vi "Get Font.vi"(0 "Font":refnum<class "Font Class.lvclass">, 7 "Font IN":T1={"Name"="STFANGSO", "Size"=12.0, "Color"=0, "Style"={"Bold"=FALSE, "Italic"=FALSE, "Underline"=FALSE, "Strikeout"=FALSE}, "Type"={"Type&direction"=enum."Select", "Embedded"=FALSE, "Encoding"=""}}, 11 "error in (no error)":errorcluster) -> (4 "Font duplicate":refnum<class "Font Class.lvclass">, 6 "Font":refnum<k24>, 8 "Font OUT":T1={"Name"="STFANGSO", "Size"=12.0, "Color"=0, "Style"={"Bold"=FALSE, "Italic"=FALSE, "Underline"=FALSE, "Strikeout"=FALSE}, "Type"={"Type&direction"=enum."Select", "Embedded"=FALSE, "Encoding"=""}}, 10 "Font Size":T2=12.0, 15 "error out":errorcluster)   [LabVIEW 2020, in "Exaprom PDF.lvlib" / "Font Class.lvclass"]
doc: "Version 1.0\nDeveloped by Jean-Marc Simard\nCopyright © 2012, Exaprom Inc.\nAll rights reserved.\nLicense: BSD\n\nWith iTextSharp 4.1.6 (http://itextsharp.sourceforge.net)\nunder Mozilla Public License Version 1.1\n(http://www.mozilla.org/MPL/MPL-1.1.html)"
uses:
  <userlib>/labview-PDF-writer-master/LV Class/Fonts Class/Font Class.lvclass
  <userlib>/labview-PDF-writer-master/Controls/Font Controls/Font complete cluster.ctl
  <userlib>/labview-PDF-writer-master/Controls/Font Controls/Font size.ctl
  <userlib>/labview-PDF-writer-master/Controls/Font Controls/Font color.ctl
  <userlib>/labview-PDF-writer-master/Controls/Font Controls/Type and encoding.ctl
  <userlib>/labview-PDF-writer-master/Controls/Text Controls/Unicode/Type and run direction.ctl
  C:/Program Files (x86)/National Instruments/LabVIEW 2020/user.lib/labview-PDF-writer-master/DLL/itextsharp.dll
  DLL/itextsharp.dll
  <userlib>/labview-PDF-writer-master/LV Class/Fonts Class/Font Class.lvclass/Font Class.ctl
  <userlib>/labview-PDF-writer-master/Exaprom PDF.lvlib
panel:
  out "NOT_EMBEDDED":bool
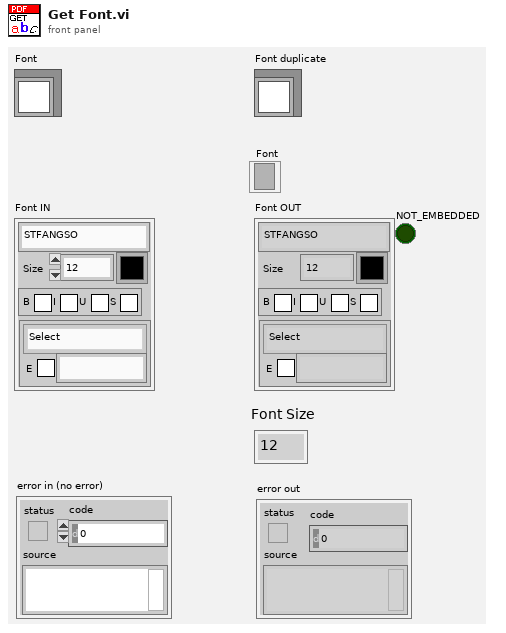
[diagram p1: front panel]
types:
  T1 = typedef "Exaprom PDF.lvlib/Font complete cluster.ctl" = cluster{"Name":string, "Size":T2, "Color":T3, "Style":cluster{"Bold":bool, "Italic":bool, "Underline":bool, "Strikeout":bool}, "Type":T4}
  T2 = typedef "Exaprom PDF.lvlib/Font size.ctl" = sgl
  T3 = typedef "Exaprom PDF.lvlib/Font color.ctl" = u32
  T4 = typedef "Exaprom PDF.lvlib/Type and encoding.ctl" = cluster{"Type&direction":T5, "Embedded":bool, "Encoding":string}
  T5 = typedef "Exaprom PDF.lvlib/Type and run direction.ctl" = enum16{"Select", "ASCII", "UTF-16", "UTF-16 (default)", "UTF-16 (LTR)", "UTF-16 (RTL)"}
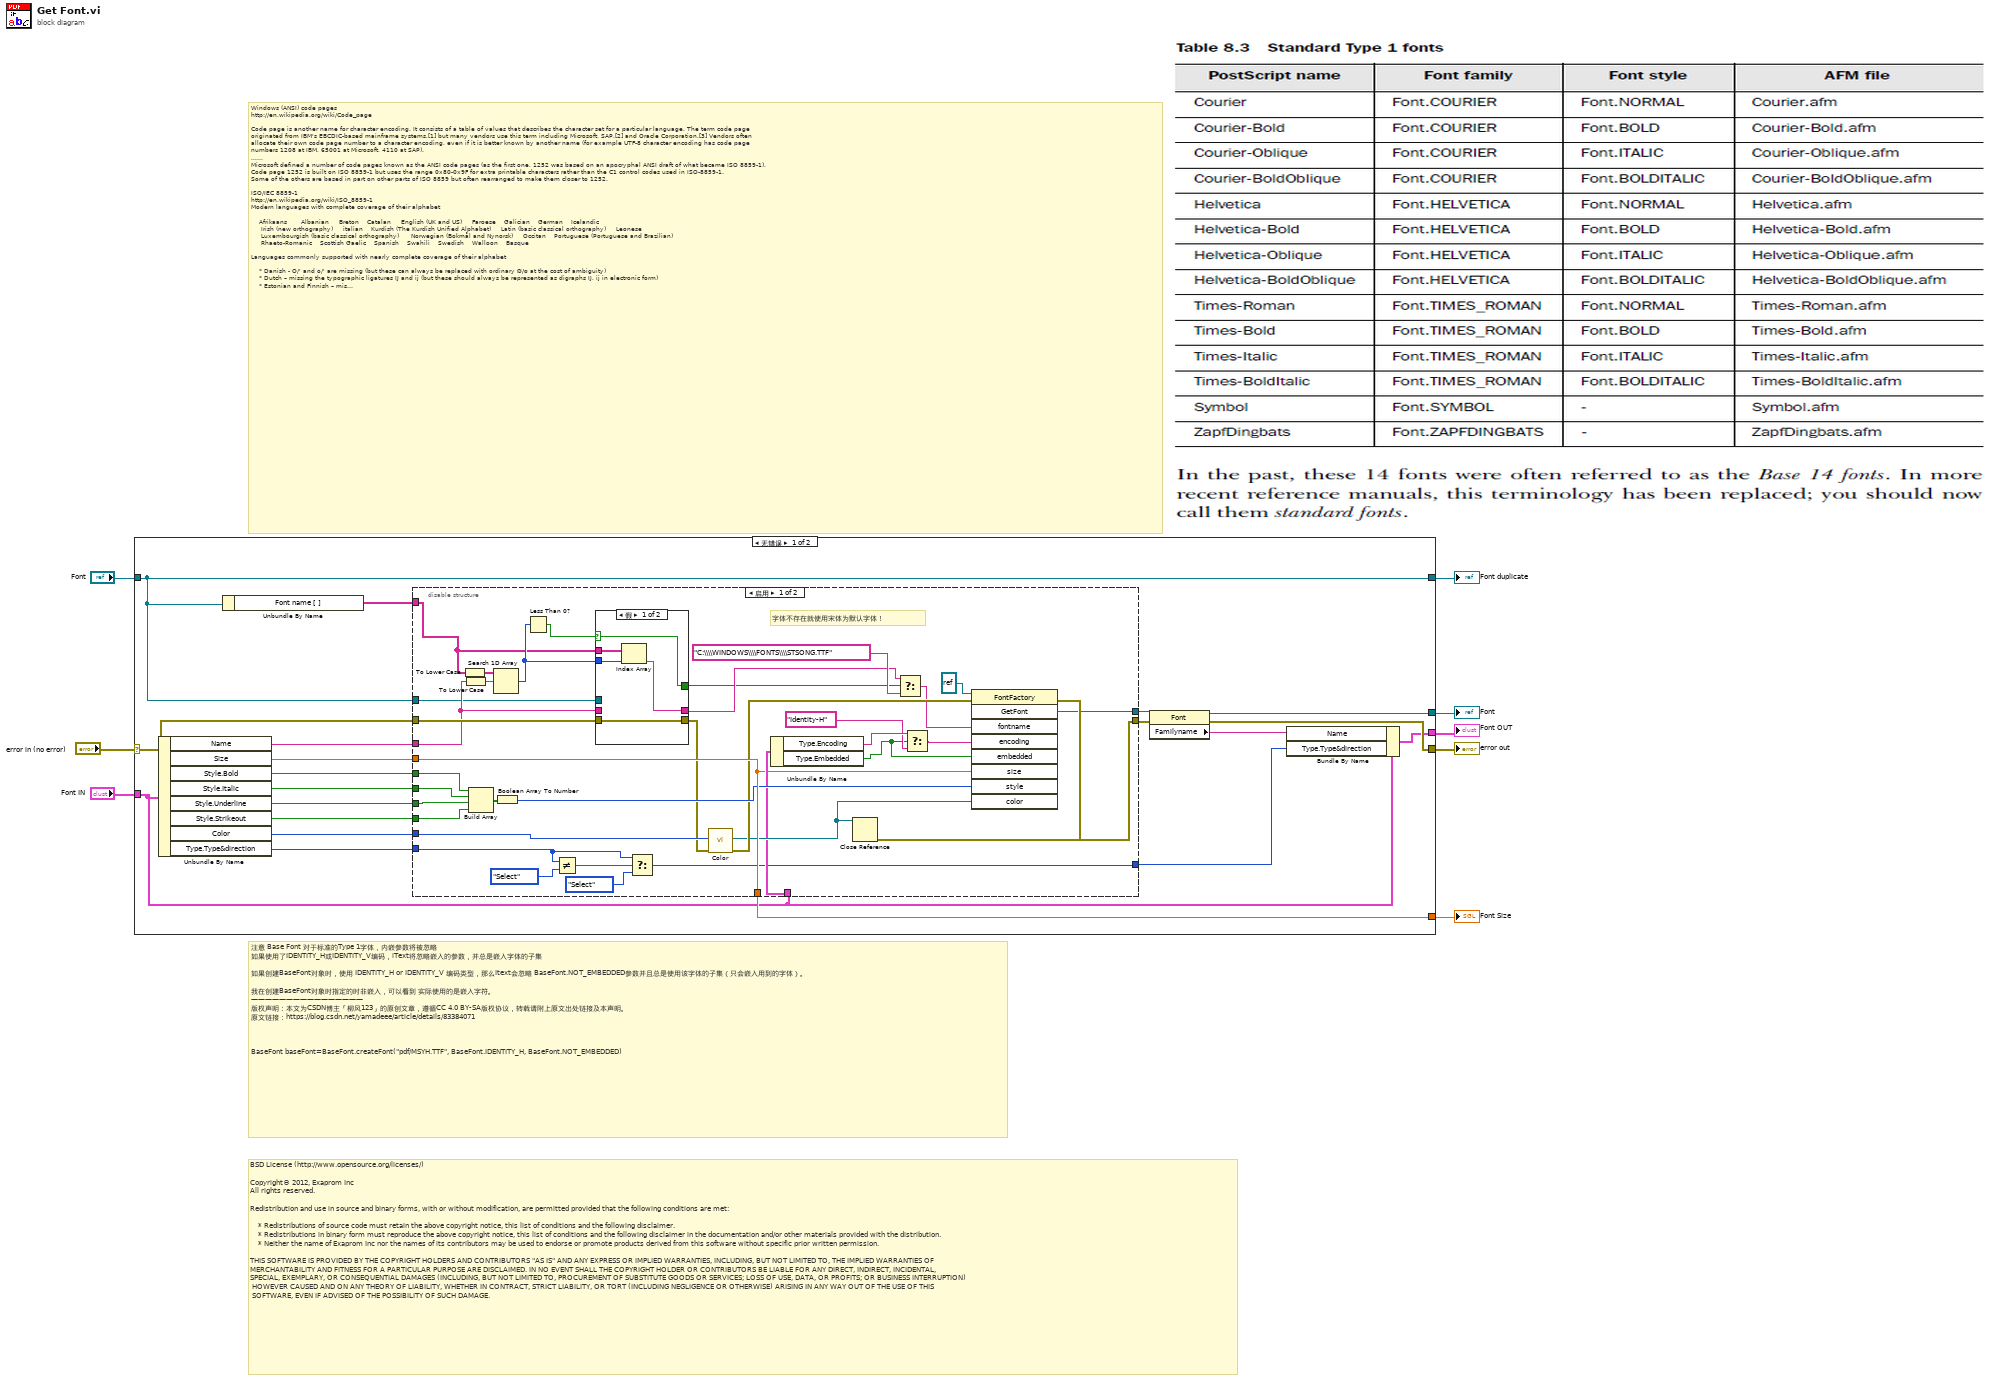
[diagram p0: block diagram]
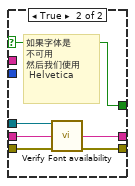
[diagram p2: hidden frame]
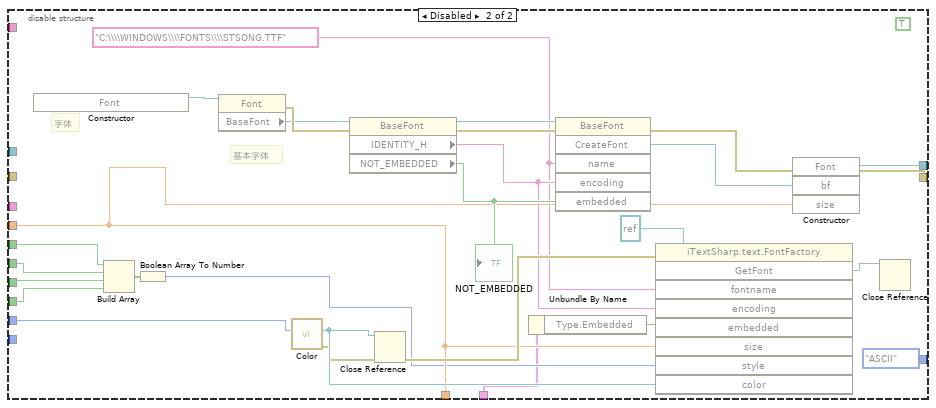
[diagram p3: hidden frame]
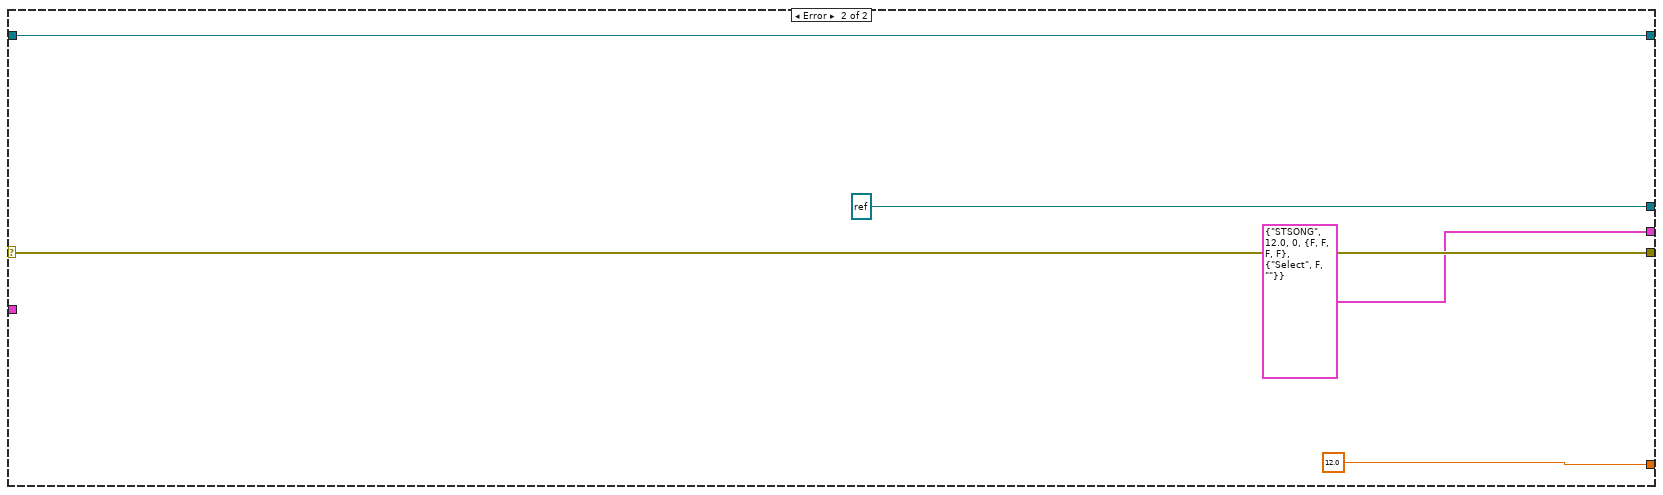
[diagram p4: hidden frame]
diagram:
  # "注意 Base Font 对于标准的Type 1字体，内嵌参数将被忽略\n如果使用了IDENTITY_H或IDENTITY_V编码，iText将忽略嵌入的参数，并总是嵌入字体的子集\n\n如果创建BaseFont对象时，使用 IDENTITY_H or IDENTITY_V 编码类型，那么Itext会忽略 BaseFont.NOT_EMBEDDED参数并且总是使用该字体的子集（只会嵌入用到的字体）。\n\n我在创建BaseFont对象时指定的时非嵌入，可以看到 实际使用的是嵌入字符。\n————————————————\n版权声明：本文为CSDN博主「柳风123」的原创文章，遵循CC 4.0 BY-SA版权协议，转载请附上原文出处链接及本声明。\n原文链接：https://blog.csdn.net/yamadeee/article/details/83384071\n\n\n\nBaseFont baseFont=BaseFont.createFont(\"pdf/MSYH.TTF\", BaseFont.IDENTITY_H, BaseFont.NOT_EMBEDDED)"
  # "Windows (ANSI) code pages\nhttp://en.wikipedia.org/wiki/Code_page\n\nCode page is another name for character encoding. It consists of a table of values that describes the character set for a particular language. The term code page\noriginated from IBM's EBCDIC-based mainframe systems,[1] but many vendors use this term including Microsoft, SAP,[2] and Oracle Corporation.[3] Vendors often\nallocate their own code page number to a character encoding, even if it is better known by another name (for example UTF-8 character encoding has code page \nnumbers 1208 at IBM, 65001 at Microsoft, 4110 at SAP).\n......\nMicrosoft defined a number of code pages known as the ANSI code pages (as the first one, 1252 was based on an apocryphal ANSI draft of what became ISO 8859-1). \nCode page 1252 is built on ISO 8859-1 but uses the range 0x80-0x9F for extra printable characters rather than the C1 control codes used in ISO-8859-1. \nSome of the others are based in part on other parts of ISO 8859 but often rearranged to make them closer to 1252.\n\nISO/IEC 8859-1\nhttp://en.wikipedia.org/wiki/ISO_8859-1\nModern languages with complete coverage of their alphabet\n\n    Afrikaans       Albanian     Breton    Catalan     English (UK and US)     Faroese    Galician    German    Icelandic\n     Irish (new orthography)     italian    Kurdish (The Kurdish Unified Alphabet)     Latin (basic classical orthography)     Leonese\n     Luxembourgish (basic classical orthography)      Norwegian (Bokmål and Nynorsk)     Occitan    Portuguese (Portuguese and Brazilian)\n     Rhaeto-Romanic    Scottish Gaelic    Spanish    Swahili    Swedish    Walloon    Basque\n\nLanguages commonly supported with nearly complete coverage of their alphabet\n\n    * Danish - O/' and o/' are missing (but these can always be replaced with ordinary Ø/ø at the cost of ambiguity)\n    * Dutch – missing the typographic ligatures IJ and ij (but these should always be represented as digraphs IJ, ij in electronic form)\n    * Estonian and Finnish – missing Š, š, Ž, ž, which can only occur in loanwords (the missing characters are often replaced by digraphs Sh, sh, Zh, zh) (Windows-1252 and ISO-8859-15 do contain these)\n    * French – missing the ligatures Œ and œ as well as the very rare Ÿ (they are generally replaced by digraphs OE and oe, and Y without the diaeresis) (Windows-1252 and ISO-8859-15 do contain these)\n    * Hungarian – missing O\", o\", U\", u\"\n    * Latin (classical language written using macrons) – missing A-, a-, E-, e-, I-, i-, O-, o-, U-, u-\n    * Welsh – missing W^, w^, Y^, y^ (ISO-8859-14 does contain these)\n    * Maori – missing A-, a-, E-, e-, I-, i-, O-, o-, U-, u-"
  # "BSD License (http://www.opensource.org/licenses/)\n\nCopyright© 2012, Exaprom Inc\nAll rights reserved.\n\nRedistribution and use in source and binary forms, with or without modification, are permitted provided that the following conditions are met:\n\n    * Redistributions of source code must retain the above copyright notice, this list of conditions and the following disclaimer.\n    * Redistributions in binary form must reproduce the above copyright notice, this list of conditions and the following disclaimer in the documentation and/or other materials provided with the distribution.\n    * Neither the name of Exaprom Inc nor the names of its contributors may be used to endorse or promote products derived from this software without specific prior written permission.\n\nTHIS SOFTWARE IS PROVIDED BY THE COPYRIGHT HOLDERS AND CONTRIBUTORS \"AS IS\" AND ANY EXPRESS OR IMPLIED WARRANTIES, INCLUDING, BUT NOT LIMITED TO, THE IMPLIED WARRANTIES OF \nMERCHANTABILITY AND FITNESS FOR A PARTICULAR PURPOSE ARE DISCLAIMED. IN NO EVENT SHALL THE COPYRIGHT HOLDER OR CONTRIBUTORS BE LIABLE FOR ANY DIRECT, INDIRECT, INCIDENTAL,\nSPECIAL, EXEMPLARY, OR CONSEQUENTIAL DAMAGES (INCLUDING, BUT NOT LIMITED TO, PROCUREMENT OF SUBSTITUTE GOODS OR SERVICES; LOSS OF USE, DATA, OR PROFITS; OR BUSINESS INTERRUPTION)\n HOWEVER CAUSED AND ON ANY THEORY OF LIABILITY, WHETHER IN CONTRACT, STRICT LIABILITY, OR TORT (INCLUDING NEGLIGENCE OR OTHERWISE) ARISING IN ANY WAY OUT OF THE USE OF THIS\n SOFTWARE, EVEN IF ADVISED OF THE POSSIBILITY OF SUCH DAMAGE."
  n1 = case shown="无错误" "error in (no error)" {
    selector: "error in (no error)" -> [w18 w106]
    tunnel: [w20 refnum<k24> refnum ("GetFont")] -> w4
    tunnel: "Font IN" -> [w15 _]
    tunnel: [w21 T2 12.0 ("Size")] -> w6
    tunnel: [w27 w106] -> w5
    tunnel: [w19 T1 {"Name"="STSONG", "Size"=12.0, "Color"=0, "Style"={"Bold"=FALSE, "Italic"=FALSE, "Underline"=FALSE, "Strikeout"=FALSE}, "Type"={"Type&direction"=enum."Select", "Embedded"=FALSE, "Encoding"=""}} ("Font OUT")] -> w3
    tunnel: "Font" -> [w10 w105]
    tunnel: [w10 w105] -> w1
    frame No Error {
      n2 = Unbundle By Name(w15) -> ("Name"=w16:string, "Size"=w21:T2, "Style.Bold"=w26:bool, "Style.Italic"=w25:bool, "Style.Underline"=w24:bool, "Style.Strikeout"=w23:bool, "Color"=w22:T3, "Type.Type&direction"=w12:T5)
      n3 = Unbundle By Name(w10) -> ("Font name [ ]"=w9:string[])
      n4 = disable-structure shown="启用" {
        disable-tunnel: w26 -> [w63 w84]
        disable-tunnel: w25 -> [w62 w83]
        disable-tunnel: w24 -> [w61 w82]
        disable-tunnel: w23 -> [w60 w81]
        disable-tunnel: w22 -> [w59 w92]
        disable-tunnel: w21 -> [w37 w86]
        disable-tunnel: w18 -> [w51 _]
        disable-tunnel: [w49 w94] -> w17
        disable-tunnel: w16 -> [w48 _]
        disable-tunnel: w15 -> [w46 w79]
        disable-tunnel: [w45 w95] -> w14
        disable-tunnel: w10 -> [w43 _]
        disable-tunnel: w12 -> [w40 _]
        disable-tunnel: [w38 Type_and_run_direction."ASCII" ("f")] -> w11
        disable-tunnel: [w37 w86] -> _
        disable-tunnel: w9 -> [w28 _]
        frame Enabled {
          # "字体不存在就使用宋体为默认字体！"
          n5 = To Lower Case(string=w28) -> (all lower case string=w54:string[])
          n6 = To Lower Case(string=w48) -> (all lower case string=w53:string)
          n7 = Build Array(w63, w62, w61, w60) -> (w64:bool[])
          n8 = Search 1D Array(1D array=w54, element=w53) -> (index of element=w47:i32)  [unwired: 1 in]
          n9 = Boolean Array To Number(Boolean array=w64) -> (number=w58:u32)
          n10 = Less Than 0?(x=w47) -> (x < 0?=w44:bool)
          n11 = Not Equal?(x=w40, y=Type_and_run_direction."Select") -> (x != y?=w41:bool)
          n12 = case shown="假" w44 {
            selector: w44 -> [w65 w70]
            tunnel: [w66 w74] -> w32
            tunnel: w48 -> [_ w75]
            tunnel: w51 -> [w69 w73]
            tunnel: [w69 w72] -> w50
            tunnel: w28 -> [w68 _]
            tunnel: w47 -> [w67 _]
            tunnel: w43 -> [_ w71]
            tunnel: [w65 w70] -> w30
            frame False {
              n13 = Index Array(array=w68, index=w67) -> (element=w66:string)
            }
            frame True {
              # "如果字体是\n不可用\n然后我们使用\n Helvetica"
              n14 = call <userlib>:"Verify Font availability.vi"("Font IN"=w71, "Font name"=w75, "error in (no error)"=w73) -> ("Font"=w74:string, "error out"=w72:errorcluster)  [unwired: 10 in, 1 out]
            }
          }
          n15 = Select(t=w40, s=w41, f=Type_and_run_direction."Select") -> (s? t:f=w38:T5)
          n16 = call <userlib>:"Color.vi"("error in (no error)"=w50, "Color"=w59) -> ("error out"=w55:errorcluster, "Color"=w52:refnum<k24>)  [unwired: 8 out]
          n17 = Unbundle By Name(w46) -> ("Type.Encoding"=w35:string, "Type.Embedded"=w29:bool)
          n18 = Select(t=w32, s=w30, f="C:\\\\WINDOWS\\\\FONTS\\\\STSONG.TTF" ("fontname")) -> (s? t:f=w31:string)
          n19 = Select(t=w35, s=w29, f="Identity-H" ("encoding")) -> (s? t:f=w36:string)
          n20 = invoke class="FontFactory" method="GetFont"(reference=refnum<k24> refnum, error in=w55, "fontname"=w31, "encoding"=w36, "embedded"=w29, "size"=w37, "style"=w58, "color"=w52) -> (error out=w56:errorcluster, "GetFont"=w45:refnum<k24>)  [unwired: 1 in, 7 out]
          n21 = Close Reference(reference=w52, error in (no error)=w56) -> (error out=w49:errorcluster)
        }
        frame Disabled {
          (unwired) TRUE
          w87 = "C:\\\\WINDOWS\\\\FONTS\\\\STSONG.TTF" ("name")
          # "基本字体"
          # "字体"
          n22 = constructor class="iTextSharp.text.Font"() -> (reference out=w100:refnum<k24>)  [unwired: 3 in, 2 out]
          n23 = Build Array(w84, w83, w82, w81) -> (w85:bool[])
          n24 = Boolean Array To Number(Boolean array=w85) -> (number=w80:u32)
          n25 = property on="属性节点" class="Font"(reference=w100) -> (error out=w101:errorcluster, "BaseFont"=w98:refnum<k24>)  [unwired: 1 in, 1 out]
          n26 = call <userlib>:"Color.vi"("Color"=w92) -> ("error out"=w90:errorcluster, "Color"=w91:refnum<k24>)  [unwired: 1 in, 8 out]
          n27 = property on="属性节点" class="BaseFont"(reference=w98, error in=w101) -> (reference out=w96:refnum<k24>, error out=w102:errorcluster, "IDENTITY_H"=w88:string, "NOT_EMBEDDED"=w97:bool)
          "NOT_EMBEDDED" <- w97
          n28 = Close Reference(reference=w91, error in (no error)=w90) -> (error out=w89:errorcluster)
          n29 = Unbundle By Name(w79) -> ("Type.Embedded"=w78:bool)
          n30 = invoke on="调用节点" class="BaseFont" method="CreateFont"(reference=w96, error in=w102, "name"=w87, "encoding"=w88, "embedded"=w97) -> (error out=w103:errorcluster, "CreateFont"=w99:refnum<k24>)  [unwired: 1 in, 4 out]
          n31 = invoke class="iTextSharp.text.FontFactory" method="GetFont"(reference=refnum<k24> refnum ("引用"), error in=w89, "fontname"=w87, "encoding"=w88, "embedded"=w78, "size"=w86, "style"=w80, "color"=w91) -> ("GetFont"=w76:refnum<k24>)  [unwired: 1 in, 8 out]
          n32 = constructor class="Font"(error in=w103, "bf"=w99, "size"=w86) -> (reference out=w95:refnum<k24>, error out=w94:errorcluster)  [unwired: 2 in, 3 out]
          n33 = Close Reference(reference=w76) -> ()  [unwired: 1 in, 1 out]
        }
      }
      n34 = property class="Font"(reference=w14, error in=w17) -> (reference out=w20:refnum<k24>, error out=w27:errorcluster, "Familyname"=w13:string)
      n35 = Bundle By Name(cluster=w15, "Name"=w13, "Type.Type&direction"=w11) -> (w19:T1)
    }
    frame Error {
    }
  }
  "error out" <- w5
  "Font" <- w4
  "Font Size" <- w6
  "Font OUT" <- w3
  "Font duplicate" <- w1
